vi "2039_2017vis FilterTargetObjects.vi"(2 "Holes Limit":i32, 3 "Lower Aspect Ratio Limit":sgl, 4 "Upper Aspect Ratio Limit":sgl, 5 "Objects":T1(array[cluster]) {"Aspect Ratio" format="%.2f"; "Orientation" format="%.2f"; "Area" format="%.2f"; "Object Center"."Y" format="%.2f"; "Object Center"."X" format="%.2f"}) -> (0 "Number of Qualified Objects":i32, 1 "Qualified Objects":T1(array[cluster]))   [LabVIEW 2016, in "2039lib.lvlib"]
uses:
  2039lib.lvlib
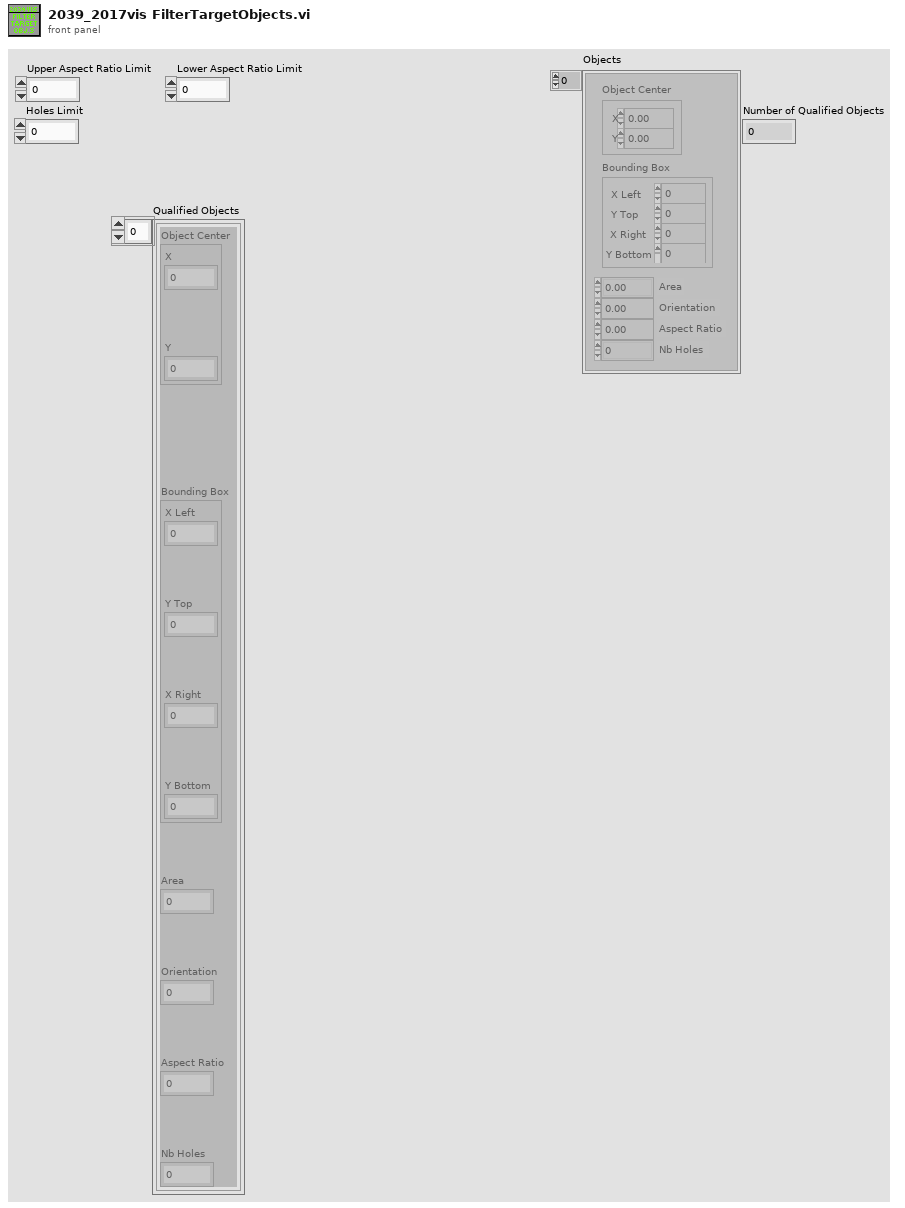
[diagram p1: front panel]
types:
  T1 = cluster{"Object Center":cluster{"X":sgl, "Y":sgl}, "Bounding Box":cluster{"X Left":i32, "Y Top":i32, "X Right":i32, "Y Bottom":i32}, "Area":sgl, "Orientation":sgl, "Aspect Ratio":sgl, "Nb Holes":i32}[]
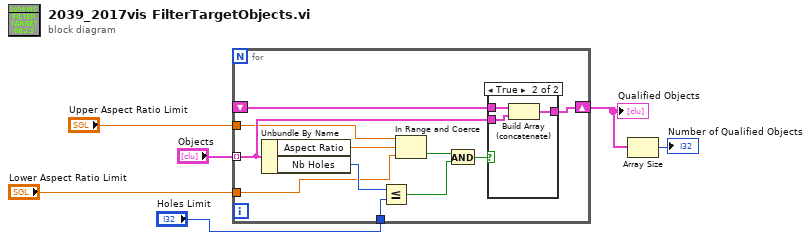
[diagram p0: block diagram]
diagram:
  n1 = for {
    tunnel: "Objects" -> [w12] mode=indexing
    shift-right: [w10] -> w5
    shift-left: _ -> [w11]
    tunnel: "Lower Aspect Ratio Limit" -> [w8]
    tunnel: "Upper Aspect Ratio Limit" -> [w9]
    tunnel: "Holes Limit" -> [w7]
    n2 = Unbundle By Name(w12) -> ("Aspect Ratio"=w17:sgl, "Nb Holes"=w16:i32)
    n3 = Less Or Equal?(x=w16, y=w7) -> (x <= y?=w14:bool)
    n4 = In Range and Coerce(upper limit=w9, x=w17, lower limit=w8) -> (In Range?=w15:bool)  [unwired: 1 out]
    n5 = And(x=w15, y=w14) -> (x .and. y?=w13:bool)
    n6 = case shown="True" w13 {
      tunnel: w12 -> [_ w21]
      tunnel: w11 -> [w18 w20]
      tunnel: [w18 w19] -> w10
      frame False {
      }
      frame True {
        n7 = Build Array (concatenate)(w20, w21) -> (w19:T1)
      }
    }
  }
  "Qualified Objects" <- w5
  n8 = Array Size(array=w5) -> (size(s)=→"Number of Qualified Objects":i32)
